vi "MindwaveCompute3Bytes.vi"(1 "INDEX":u8, 2 "RAW_ARRAY":u8[](array[numeric]) format="%x") -> (0 "RAW_VALUE":u32 format="%x")   [LabVIEW 2011, in "Neurosky.lvlib"]
uses:
  Users/Isaias/Documents/GitHub/Neurosky/Neurosky.lvlib
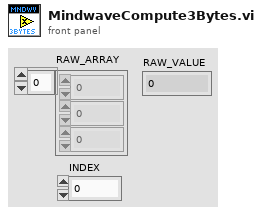
[diagram p1: front panel]
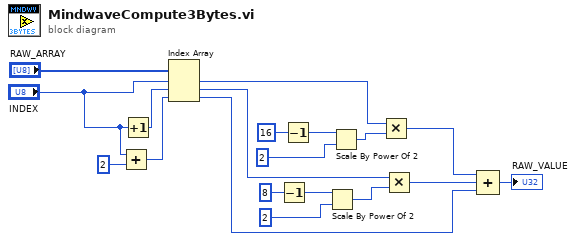
[diagram p0: block diagram]
diagram:
  n1 = Add(x="INDEX", y=u8 2) -> (x+y=w15:u8)
  n2 = Increment(x="INDEX") -> (x+1=w18:u8)
  n3 = Index Array(array="RAW_ARRAY", index #1="INDEX", index #2=w18, index #3=w15) -> (element #1=w10:u8, element #2=w6:u8, element #3=w2:u8)
  n4 = Decrement(x=u8 8 ("y")) -> (x-1=w8:u8)
  n5 = Decrement(x=u8 16 ("y")) -> (x-1=w13:u8)
  n6 = Scale By Power Of 2(n=w8, x=u16 2 ("y")) -> (x*2^n=w5:u16)
  n7 = Scale By Power Of 2(n=w13, x=u32 2 ("y")) -> (x*2^n=w11:u32)
  n8 = Multiply(x=w10, y=w11) -> (x*y=w4:u32)
  n9 = Multiply(x=w6, y=w5) -> (x*y=w3:u16)
  n10 = Compound Arithmetic op=ADD(w4, w3, w2) -> (→"RAW_VALUE":u32)
